vi "CreateNewSystemDefinition.vi"(8 "error in":errorcluster, 10 "OS (Windows)":string, 11 "System Definition Name":string) -> (0 "error out":errorcluster, 3 "System Definition Path":path)   [LabVIEW 2017, in "VeriStandTestUtilities.lvlib"]
uses:
  VeriStandTestUtilities.lvlib
  NationalInstruments.VeriStand.SystemDefinitionAPI
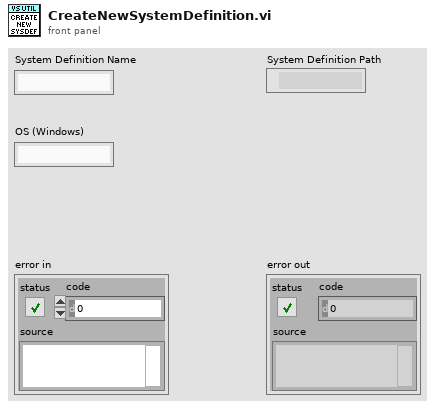
[diagram p1: front panel]
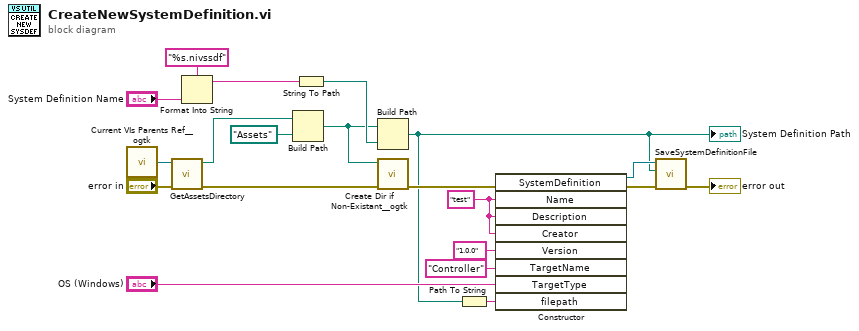
[diagram p0: block diagram]
diagram:
  w15 = "test" ("Name")
  n1 = call <userlib>:"Current VIs Parents Ref__ogtk.vi"() -> ("Calling VI's Reference"=w5:refnum<vi>)  [unwired: 2 in]
  n2 = call "GetAssetsDirectory.vi"("error in"="error in", "test VI refnum"=w5) -> ("error out"=w6:errorcluster, "assets dir"=w4:path)  [unwired: 8 in]
  n3 = Format Into String(format string="%s.nivssdf", "System Definition Name") -> (resulting string=w1:string)  [unwired: 2 in, 1 out]
  n4 = Build Path(base path=w4, name or relative path=path "Assets") -> (appended path=w17:path)
  n5 = String To Path(string=w1) -> (path=w18:path)
  n6 = Build Path(base path=w17, name or relative path=w18) -> (appended path=w9:path)
  "System Definition Path" <- w9
  n7 = call <userlib>:"Create Dir if Non-Existant__ogtk.vi"("error in (no error)"=w6, "Directory Path"=w17) -> ("error out"=w16:errorcluster)  [unwired: 7 in, 2 out]
  n8 = Path To String(path=w9) -> (string=w11:string)
  n9 = constructor class="SystemDefinition"(error in=w16, "Name"=w15, "Description"=w15, "Creator"=w15, "Version"="1.0.0", "TargetName"="Controller", "TargetType"="OS (Windows)", "filepath"=w11) -> (reference out=w10:refnum<k24>, error out=w20:errorcluster)  [unwired: 2 in, 8 out]
  n10 = call "SaveSystemDefinitionFile.vi"("error in (no error)"=w20, "System Definition File in"=w9, "System Definition Reference in"=w10) -> ("error out"=→"error out":errorcluster)  [unwired: 7 in, 1 out]
